vi "Set Value Variant.vi"(8 "error in (no error)":errorcluster, 10 "value":variant, 11 "value pointer in":i64) -> (0 "error out":errorcluster, 2 "value out":variant, 3 "value pointer out":i64)   [LabVIEW 2020, in "Value.lvlib"]
uses:
  Value.lvlib
  cceb9e4b-eb75-48e8-aa55-ce9bdc72e988.vi
  a45a0ea4-a1a3-4c44-a2d0-bd9ac2191226.vi
  c2285a35-9ffd-4e7b-9c27-aea24fb1581d.vi
  8f9649cc-7f21-4ef7-860a-133741f03507.vi
  9a7adfbc-dfd7-46c4-b075-4f0440b83174.vi
  f3df2b06-57d5-4a32-8a6e-a93eab4b8334.vi
  1bea9b6c-c326-4b2e-8e3d-45bf733a9c38.vi
  e383973c-90af-4a51-a4c7-5bbe8c763ef6.vi
  d9fbc47b-4e38-408d-93dd-f03e8c927dfc.vi
  f8e0b90b-c4e6-43ce-b49d-bcdb382c13bb.vi
  878da8d4-af84-4ac8-b8bd-4e3d6f536ca0.vi
  1aa6b969-7b68-4eb2-b836-e13a600a071e.vi
  22b99ade-ebf6-47b9-88b0-a2a84584e77c.vi
  0ecc3a10-4d88-4a3f-8e2b-6d81b1eb2788.vi
  7938dc55-06bb-4f46-98b4-31ec94e48f5a.vi
  9cf4c5a1-706a-4248-a3ee-b4c9f4ce04b3.vi
  17bcbbb4-445b-4ae2-9ca0-bb438421ceb4.vi
  ae889fb9-670a-49f8-b5e5-a0c16fe27676.vi
  76e53dd5-f0c3-4a89-968d-82371d9cf6ec.vi
  bc742d90-07da-41a2-bb0a-7e7b2f4baedd.vi
  9c6bba7f-697c-4d5e-a550-b75ffba85a50.vi
  d17b89b1-25de-4b77-9841-199634659aba.vi
  02c85caf-8b62-432b-a175-5fdc5c038fcc.vi
  db2778e5-0a0b-476e-a616-76c34d6078df.vi
  5a5bdb7c-77ef-45fb-97e8-dbe02cadd076.vi
  03112d84-5c9b-4772-aceb-1428f387a576.vi
  b370053f-91cb-4be5-8525-cb241afcd6fe.vi
  21acc165-9bb3-46db-a53e-93d4eb7e31ab.vi
  a549df2c-920d-4323-ba7c-d4da420400e8.vi
  6d74252b-ad3a-45a7-9484-b3c05cdeac0b.vi
  79192ce2-8dd6-4a70-8822-a4eb65a6aaee.vi
  8a659153-4bf4-400b-b716-4e15b1f2a15f.vi
  1431eaa6-23a1-45b9-a4a3-2693041a1402.vi
  8366b1b6-5195-4a32-8846-ef1dc1edc039.vi
  05adf883-15cd-45cb-9d7e-7746134da8fa.vi
  522d9441-c019-479c-9fbf-718d84229053.vi
  2414d7e0-05f5-4190-ab07-d4c7ba67c6a6.vi
  16fc2f7d-2f3d-48d7-828e-6f1655900f08.vi
  efa8a1d7-3bed-4705-901c-3918d28cffa5.vi
  be3d0229-b834-4748-a57b-b2038c1c1ccb.vi
  26f11cd7-ec94-4004-9a33-110acaed2e3e.vi
  270ebb12-d336-49d8-bcbc-e0196ad89af1.vi
  cc62e3b5-8986-4e79-a38c-535dac47f5c9.vi
  6a645410-e7ef-4ed8-b58d-cdb6402696f2.vi
  21c48d27-f92c-4ff3-9f7e-da22303d9520.vi
  71c37fb2-0984-443b-b7b1-928344430237.vi
  0dfc8336-85bc-4349-aa6f-77eea7d3ae68.vi
  d4fece01-f7e1-4bf9-a8a9-9bacda043edb.vi
  <vilib>/Utility/error.llb/Clear Errors.vi
  <vilib>/Utility/Data Type/Get Type Information.vi
  <vilib>/Utility/Data Type/Get Array Information.vi
  <vilib>/Utility/error.llb/Error Cluster From Error Code.vi
  Get Library Path.vi
  <vilib>/ErrorRing/Error Ring.xnode
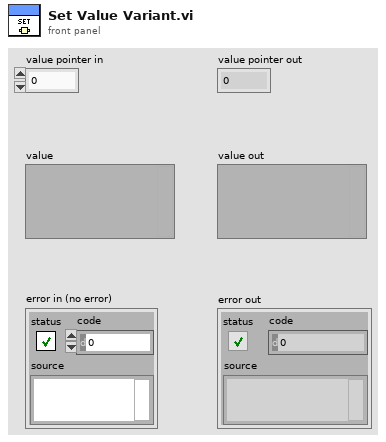
[diagram p1: front panel]
types:
  T1 = typedef "Value.lvlib/TypeCode.ctl" = enum8{"Null", "Bool", "BoolA", "Int8", "Int8A", "Int16", "Int16A", "Int32", "Int32A", "Int64", "Int64A", "UInt8", "UInt8A", "UInt16", "UInt16A", "UInt32", "UInt32A", "UInt64", "UInt64A", "Float32", "Float32A", "Float64", "Float64A", "String", "StringA", "Struct", "StructA", "Union", "UnionA", "Any", "AnyA"}
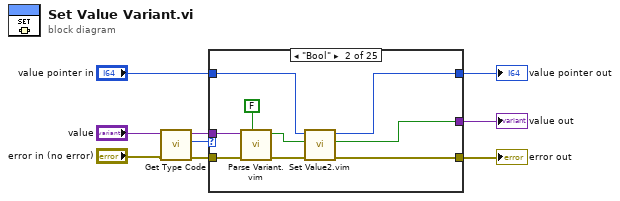
[diagram p0: block diagram]
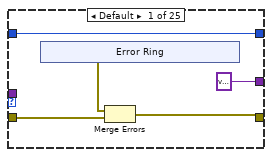
[diagram p2: hidden frame]
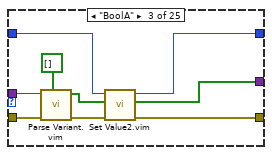
[diagram p3: hidden frame]
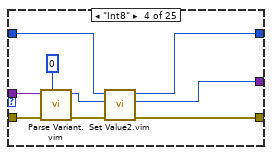
[diagram p4: hidden frame]
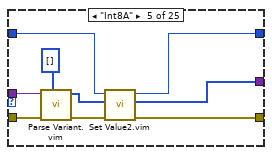
[diagram p5: hidden frame]
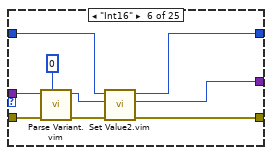
[diagram p6: hidden frame]
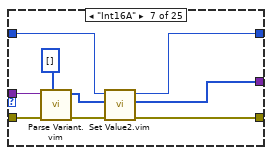
[diagram p7: hidden frame]
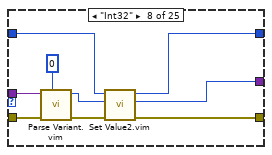
[diagram p8: hidden frame]
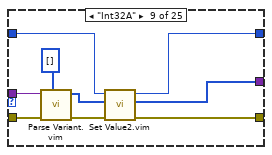
[diagram p9: hidden frame]
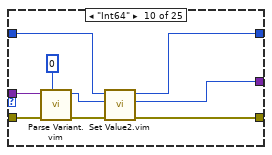
[diagram p10: hidden frame]
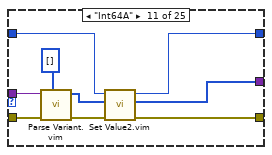
[diagram p11: hidden frame]
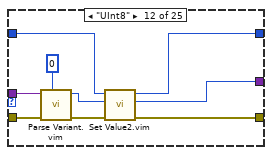
[diagram p12: hidden frame]
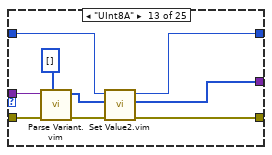
[diagram p13: hidden frame]
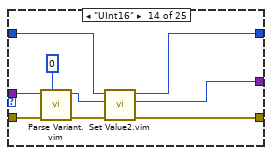
[diagram p14: hidden frame]
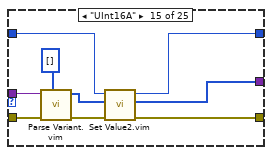
[diagram p15: hidden frame]
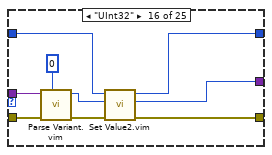
[diagram p16: hidden frame]
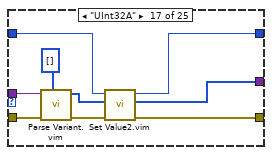
[diagram p17: hidden frame]
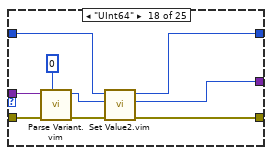
[diagram p18: hidden frame]
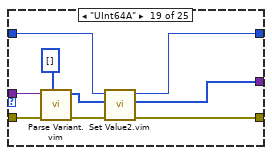
[diagram p19: hidden frame]
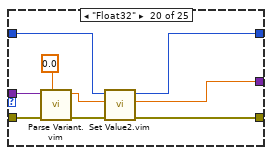
[diagram p20: hidden frame]
diagram:
  n1 = call "Get Type Code.vi"("error in (no error)"="error in (no error)", "value"="value") -> ("error out"=w7:errorcluster, "type code"=w9:T1, "value dup"=w8:variant)  [unwired: 5 in]
  n2 = case shown="\"Bool\"" w9 {
    tunnel: [w13 w24 w34 w43 w52 w61 w70 w79 w88 w97 w107 w115 w124 w133 w142 w151 w160 w169 w178 w187 w196 w205 w214 w223 w232] -> w1
    tunnel: w7 -> [w14 w27 w36 w45 w54 w63 w72 w81 w90 w99 w108 w117 w126 w135 w144 w153 w162 w171 w180 w189 w198 w207 w216 w225 w234]
    tunnel: [w10 w22 w32 w42 w50 w59 w68 w77 w86 w95 w105 w113 w122 w132 w140 w149 w159 w167 w176 w185 w194 w203 w212 w221 w230] -> w3
    tunnel: w8 -> [_ w21 w31 w41 w49 w58 w67 w76 w85 w94 w104 w112 w121 w131 w139 w148 w158 w166 w175 w184 w193 w202 w211 w220 w229]
    tunnel: [variant w20 w29 w39 w47 w56 w65 w74 w83 w92 w102 w110 w119 w129 w137 w146 w156 w164 w173 w182 w191 w200 w209 w218 w227] -> w2
    tunnel: "value pointer in" -> [w10 w19 w28 w38 w46 w55 w64 w73 w82 w91 w100 w109 w118 w128 w136 w145 w155 w163 w172 w181 w190 w199 w208 w217 w226]
    frame Default {
      n3 = xnode "Error Ring"() -> ("error out"=w12:errorcluster)
      n4 = Merge Errors(w12, w14) -> (w13:errorcluster)
    }
    frame "Bool" {
      n5 = call "Parse Variant.vim"("default"=FALSE, "error in (no error)"=w27, "value"=w21) -> ("error out"=w25:errorcluster, "value out"=w23:bool)  [unwired: 7 in]
      n6 = call "Set Value2.vim"("error in"=w25, "value"=w23, "value pointer in"=w19) -> ("error out"=w24:errorcluster, "value out"=w20:bool, "value pointer out"=w22:i64)  [unwired: 6 in]
    }
    frame "BoolA" {
      n7 = call "Parse Variant.vim"("default"=bool[] [], "error in (no error)"=w36, "value"=w31) -> ("error out"=w35:errorcluster, "value out"=w33:bool[])  [unwired: 7 in]
      n8 = call "Set Value2.vim"("error in"=w35, "value"=w33, "value pointer in"=w28) -> ("error out"=w34:errorcluster, "value out"=w29:bool[], "value pointer out"=w32:i64)  [unwired: 6 in]
    }
    frame "Int8" {
      n9 = call "Parse Variant.vim"("default"=i8 0, "error in (no error)"=w45, "value"=w41) -> ("error out"=w44:errorcluster, "value out"=w37:i8)  [unwired: 7 in]
      n10 = call "Set Value2.vim"("error in"=w44, "value"=w37, "value pointer in"=w38) -> ("error out"=w43:errorcluster, "value out"=w39:i8, "value pointer out"=w42:i64)  [unwired: 6 in]
    }
    frame "Int8A" {
      n11 = call "Parse Variant.vim"("default"=i8[] [], "error in (no error)"=w54, "value"=w49) -> ("error out"=w53:errorcluster, "value out"=w51:i8[])  [unwired: 7 in]
      n12 = call "Set Value2.vim"("error in"=w53, "value"=w51, "value pointer in"=w46) -> ("error out"=w52:errorcluster, "value out"=w47:i8[], "value pointer out"=w50:i64)  [unwired: 6 in]
    }
    frame "Int16" {
      n13 = call "Parse Variant.vim"("default"=i16 0, "error in (no error)"=w63, "value"=w58) -> ("error out"=w62:errorcluster, "value out"=w60:i16)  [unwired: 7 in]
      n14 = call "Set Value2.vim"("error in"=w62, "value"=w60, "value pointer in"=w55) -> ("error out"=w61:errorcluster, "value out"=w56:i16, "value pointer out"=w59:i64)  [unwired: 6 in]
    }
    frame "Int16A" {
      n15 = call "Parse Variant.vim"("default"=i16[] [], "error in (no error)"=w72, "value"=w67) -> ("error out"=w71:errorcluster, "value out"=w69:i16[])  [unwired: 7 in]
      n16 = call "Set Value2.vim"("error in"=w71, "value"=w69, "value pointer in"=w64) -> ("error out"=w70:errorcluster, "value out"=w65:i16[], "value pointer out"=w68:i64)  [unwired: 6 in]
    }
    frame "Int32" {
      n17 = call "Parse Variant.vim"("default"=0, "error in (no error)"=w81, "value"=w76) -> ("error out"=w80:errorcluster, "value out"=w78:i32)  [unwired: 7 in]
      n18 = call "Set Value2.vim"("error in"=w80, "value"=w78, "value pointer in"=w73) -> ("error out"=w79:errorcluster, "value out"=w74:i32, "value pointer out"=w77:i64)  [unwired: 6 in]
    }
    frame "Int32A" {
      n19 = call "Parse Variant.vim"("default"=i32[] [], "error in (no error)"=w90, "value"=w85) -> ("error out"=w89:errorcluster, "value out"=w87:i32[])  [unwired: 7 in]
      n20 = call "Set Value2.vim"("error in"=w89, "value"=w87, "value pointer in"=w82) -> ("error out"=w88:errorcluster, "value out"=w83:i32[], "value pointer out"=w86:i64)  [unwired: 6 in]
    }
    frame "Int64" {
      n21 = call "Parse Variant.vim"("default"=i64 0, "error in (no error)"=w99, "value"=w94) -> ("error out"=w98:errorcluster, "value out"=w96:i64)  [unwired: 7 in]
      n22 = call "Set Value2.vim"("error in"=w98, "value"=w96, "value pointer in"=w91) -> ("error out"=w97:errorcluster, "value out"=w92:i64, "value pointer out"=w95:i64)  [unwired: 6 in]
    }
    frame "Int64A" {
      n23 = call "Parse Variant.vim"("default"=i64[] [], "error in (no error)"=w108, "value"=w104) -> ("error out"=w101:errorcluster, "value out"=w106:i64[])  [unwired: 7 in]
      n24 = call "Set Value2.vim"("error in"=w101, "value"=w106, "value pointer in"=w100) -> ("error out"=w107:errorcluster, "value out"=w102:i64[], "value pointer out"=w105:i64)  [unwired: 6 in]
    }
    frame "UInt8" {
      n25 = call "Parse Variant.vim"("default"=u8 0, "error in (no error)"=w117, "value"=w112) -> ("error out"=w116:errorcluster, "value out"=w114:u8)  [unwired: 7 in]
      n26 = call "Set Value2.vim"("error in"=w116, "value"=w114, "value pointer in"=w109) -> ("error out"=w115:errorcluster, "value out"=w110:u8, "value pointer out"=w113:i64)  [unwired: 6 in]
    }
    frame "UInt8A" {
      n27 = call "Parse Variant.vim"("default"=u8[] [], "error in (no error)"=w126, "value"=w121) -> ("error out"=w125:errorcluster, "value out"=w123:u8[])  [unwired: 7 in]
      n28 = call "Set Value2.vim"("error in"=w125, "value"=w123, "value pointer in"=w118) -> ("error out"=w124:errorcluster, "value out"=w119:u8[], "value pointer out"=w122:i64)  [unwired: 6 in]
    }
    frame "UInt16" {
      n29 = call "Parse Variant.vim"("default"=u16 0, "error in (no error)"=w135, "value"=w131) -> ("error out"=w134:errorcluster, "value out"=w127:u16)  [unwired: 7 in]
      n30 = call "Set Value2.vim"("error in"=w134, "value"=w127, "value pointer in"=w128) -> ("error out"=w133:errorcluster, "value out"=w129:u16, "value pointer out"=w132:i64)  [unwired: 6 in]
    }
    frame "UInt16A" {
      n31 = call "Parse Variant.vim"("default"=u16[] [], "error in (no error)"=w144, "value"=w139) -> ("error out"=w143:errorcluster, "value out"=w141:u16[])  [unwired: 7 in]
      n32 = call "Set Value2.vim"("error in"=w143, "value"=w141, "value pointer in"=w136) -> ("error out"=w142:errorcluster, "value out"=w137:u16[], "value pointer out"=w140:i64)  [unwired: 6 in]
    }
    frame "UInt32" {
      n33 = call "Parse Variant.vim"("default"=u32 0, "error in (no error)"=w153, "value"=w148) -> ("error out"=w152:errorcluster, "value out"=w150:u32)  [unwired: 7 in]
      n34 = call "Set Value2.vim"("error in"=w152, "value"=w150, "value pointer in"=w145) -> ("error out"=w151:errorcluster, "value out"=w146:u32, "value pointer out"=w149:i64)  [unwired: 6 in]
    }
    frame "UInt32A" {
      n35 = call "Parse Variant.vim"("default"=u32[] [], "error in (no error)"=w162, "value"=w158) -> ("error out"=w161:errorcluster, "value out"=w154:u32[])  [unwired: 7 in]
      n36 = call "Set Value2.vim"("error in"=w161, "value"=w154, "value pointer in"=w155) -> ("error out"=w160:errorcluster, "value out"=w156:u32[], "value pointer out"=w159:i64)  [unwired: 6 in]
    }
    frame "UInt64" {
      n37 = call "Parse Variant.vim"("default"=u64 0, "error in (no error)"=w171, "value"=w166) -> ("error out"=w170:errorcluster, "value out"=w168:u64)  [unwired: 7 in]
      n38 = call "Set Value2.vim"("error in"=w170, "value"=w168, "value pointer in"=w163) -> ("error out"=w169:errorcluster, "value out"=w164:u64, "value pointer out"=w167:i64)  [unwired: 6 in]
    }
    frame "UInt64A" {
      n39 = call "Parse Variant.vim"("default"=u64[] [], "error in (no error)"=w180, "value"=w175) -> ("error out"=w179:errorcluster, "value out"=w177:u64[])  [unwired: 7 in]
      n40 = call "Set Value2.vim"("error in"=w179, "value"=w177, "value pointer in"=w172) -> ("error out"=w178:errorcluster, "value out"=w173:u64[], "value pointer out"=w176:i64)  [unwired: 6 in]
    }
    frame "Float32" {
      n41 = call "Parse Variant.vim"("default"=sgl 0.0, "error in (no error)"=w189, "value"=w184) -> ("error out"=w188:errorcluster, "value out"=w186:sgl)  [unwired: 7 in]
      n42 = call "Set Value2.vim"("error in"=w188, "value"=w186, "value pointer in"=w181) -> ("error out"=w187:errorcluster, "value out"=w182:sgl, "value pointer out"=w185:i64)  [unwired: 6 in]
    }
    frame "Float64" {
      n43 = call "Parse Variant.vim"("default"=0.0, "error in (no error)"=w198, "value"=w193) -> ("error out"=w197:errorcluster, "value out"=w195:dbl)  [unwired: 7 in]
      n44 = call "Set Value2.vim"("error in"=w197, "value"=w195, "value pointer in"=w190) -> ("error out"=w196:errorcluster, "value out"=w191:dbl, "value pointer out"=w194:i64)  [unwired: 6 in]
    }
    frame "Float32A" {
      n45 = call "Parse Variant.vim"("default"=sgl[] [], "error in (no error)"=w207, "value"=w202) -> ("error out"=w206:errorcluster, "value out"=w204:sgl[])  [unwired: 7 in]
      n46 = call "Set Value2.vim"("error in"=w206, "value"=w204, "value pointer in"=w199) -> ("error out"=w205:errorcluster, "value out"=w200:sgl[], "value pointer out"=w203:i64)  [unwired: 6 in]
    }
    frame "Float64A" {
      n47 = call "Parse Variant.vim"("default"=dbl[] [], "error in (no error)"=w216, "value"=w211) -> ("error out"=w215:errorcluster, "value out"=w213:dbl[])  [unwired: 7 in]
      n48 = call "Set Value2.vim"("error in"=w215, "value"=w213, "value pointer in"=w208) -> ("error out"=w214:errorcluster, "value out"=w209:dbl[], "value pointer out"=w212:i64)  [unwired: 6 in]
    }
    frame "String" {
      n49 = call "Parse Variant.vim"("default"="", "error in (no error)"=w225, "value"=w220) -> ("error out"=w224:errorcluster, "value out"=w222:string)  [unwired: 7 in]
      n50 = call "Set Value2.vim"("error in"=w224, "value"=w222, "value pointer in"=w217) -> ("error out"=w223:errorcluster, "value out"=w218:string, "value pointer out"=w221:i64)  [unwired: 6 in]
    }
    frame "StringA" {
      n51 = call "Parse Variant.vim"("default"=string[] [], "error in (no error)"=w234, "value"=w229) -> ("error out"=w233:errorcluster, "value out"=w231:string[])  [unwired: 7 in]
      n52 = call "Set Value2.vim"("error in"=w233, "value"=w231, "value pointer in"=w226) -> ("error out"=w232:errorcluster, "value out"=w227:string[], "value pointer out"=w230:i64)  [unwired: 6 in]
    }
  }
  "value pointer out" <- w3
  "value out" <- w2
  "error out" <- w1
